vi "SavePicture.vi"(6 "File Path":path, 8 "Image Pixels (U16)":u16[][](array[numeric])) -> (0 "error out":errorcluster)   [LabVIEW 2014]
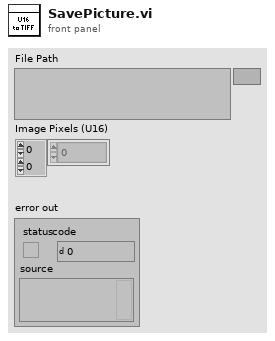
[diagram p1: front panel]
types:
  T1 = typedef "Image Type" = u32
  T2 = typedef "IMAQ Image.ctl" = refnum<image>
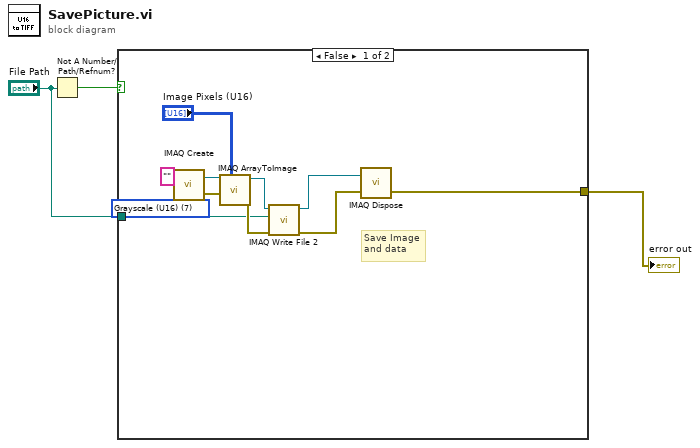
[diagram p0: block diagram]
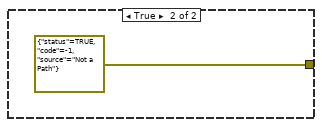
[diagram p2: hidden frame]
diagram:
  n1 = Not A Number/Path/Refnum?(number/path/refnum="File Path") -> (NaN/Path/Refnum?=w3:bool)
  n2 = case shown="False" w3 {
    tunnel: [w6 errorcluster {"status"=TRUE, "code"=-1, "source"="Not a Path"} ("error out")] -> w2
    tunnel: "File Path" -> [w5 _]
    frame False {
      w4 = T1 7 items=["Grayscale (U8)", "Grayscale (I16)", "Grayscale (SGL)", "Complex (CSG)", "RGB (U32)", "HSL (U32)", "RGB (U64)", "Grayscale (U16)"] ("Image Type")
      # "Save Image\nand data"
      n3 = call "IMAQ Create"("Image Name"="", "Image Type"=w4) -> ("New Image"=w11:T2, "error out"=w12:errorcluster)  [unwired: 3 in]
      n4 = call "IMAQ ArrayToImage"("Image Pixels (U16)"="Image Pixels (U16)", "error in (no error)"=w12, "Image"=w11) -> ("error out"=w9:errorcluster, "Image Out"=w10:T2)  [unwired: 7 in]
      n5 = call-poly "IMAQ Write File 2"("error in (no error)"=w9, "File Path"=w5, "Image"=w10) -> ("error out"=w13:errorcluster, "Image Out (duplicate)"=w14:T2)  [unwired: 7 in]
      n6 = call "IMAQ Dispose"("Image"=w14, "error in (no error)"=w13) -> ("error out"=w6:errorcluster)  [unwired: 4 in]
    }
    frame True {
    }
  }
  "error out" <- w2
